vi "Initialize.vi"(7 "menu ref":refnum<k9>, 8 "error in":errorcluster, 9 "dynamic event queue reference":T1, 10 "User Interface Control Reference":refnum<queue>, 11 "User Event Control Reference":refnum<queue>) -> (0 "error out":errorcluster)   [LabVIEW 2011]
uses:
  Controls/Dynamic Event Queue Reference.ctl
  Controls/User Interface Control.ctl
  Controls/User Interface Action.ctl
  Controls/User Event Control.ctl
  Controls/User Event Action.ctl
  Functional Globals/General Flags.ctl
  Functional Globals/User Interface Global Action.ctl
  Error Handling/Error Module Action.ctl
  Functional Globals/Pulse Parameters.ctl
  Modules/Menu/Menu Action.ctl
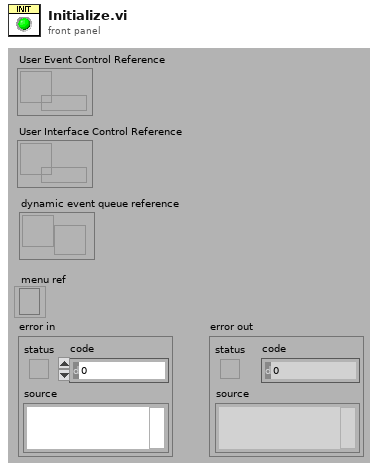
[diagram p1: front panel]
types:
  T1 = typedef "Dynamic Event Queue Reference.ctl" = refnum<user-event>
  T2 = typedef "General Flags.ctl" = enum16{"Initialize", "Set Abort Flag", "Get Abort Flag"}
  T3 = typedef "User Interface Global Action.ctl" = enum16{"Initialize", "Update UI", "Stop"}
  T4 = typedef "Error Module Action.ctl" = enum16{"Initialize", "Handle Errors", "Report Errors"}
  T5 = typedef "Pulse Parameters.ctl" = enum16{"Initialize", "Set T1 Pulse Settings", "Set 90 Degree Pulse Settings", "Set CPMG Pulse Settings", "Get T1 Settings", "Get CPMG Settings", "Get 90 Degree Settings"}
  T6 = typedef "Menu Action.ctl" = enum16{"Initialize", "Insert Item", "Remove Item", "Set Checked Item", "Get Checked Item", "Get Item Index", "Item Present?", "Stop"}
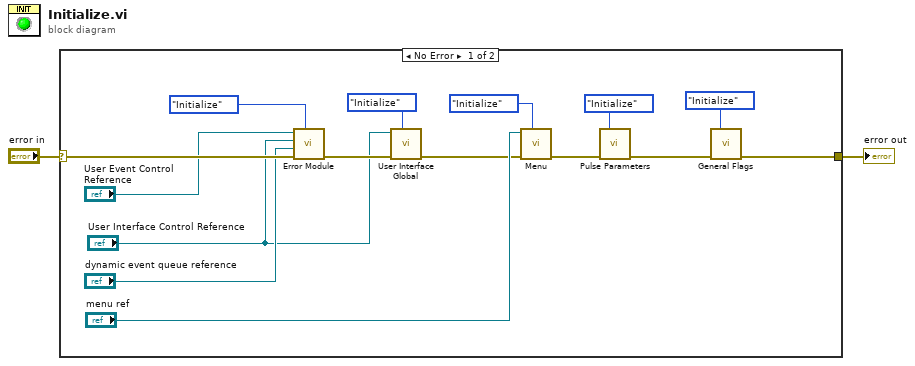
[diagram p0: block diagram]
diagram:
  n1 = case shown="No Error" "error in" {
    selector: "error in" -> [w17 w18]
    tunnel: [w3 w18] -> w1
    frame No Error {
      n2 = call "Error Module.vi"("command (handle errors)"=Error_Module_Action."Initialize", "error in"=w17, "dynamic event queue reference"="dynamic event queue reference", "User Interface Control Reference"="User Interface Control Reference", "User Event Control Reference"="User Event Control Reference") -> ("error out"=w9:errorcluster)  [unwired: 5 in, 1 out]
      n3 = call "User Interface Global.vi"("command (Update UI)"=User_Interface_Global_Action."Initialize", "error in"=w9, "user interface queue reference"="User Interface Control Reference") -> ("error out"=w8:errorcluster)  [unwired: 8 in]
      n4 = call "Menu.vi"("action"=Menu_Action."Initialize" ("Menu"), "error in"=w8, "menu reference"="menu ref") -> ("error out"=w12:errorcluster)  [unwired: 5 in, 3 out]
      n5 = call "Pulse Parameters.vi"("action"=Pulse_Parameters."Initialize", "error in"=w12) -> ("error out"=w4:errorcluster)  [unwired: 6 in, 7 out]
      n6 = call "General Flags.vi"("action"=General_Flags."Initialize" ("Action"), "error in"=w4) -> ("error out"=w3:errorcluster)  [unwired: 12 in, 1 out]
    }
    frame Error {
    }
  }
  "error out" <- w1
